vi "Can_Add.vi"(8 "error in (no error)":errorcluster, 11 "IB_Tree_Item_Proj_Folder in":refnum<class "IB_Tree_Item_Proj_Folder.lvclass">) -> (0 "error out":errorcluster, 2 "can add?":bool, 3 "IB_Tree_Item_Proj_Folder out":refnum<class "IB_Tree_Item_Proj_Folder.lvclass">)   [LabVIEW 2020, in "IB_Tree_Item_Proj_Folder.lvclass"]
uses:
  <vilib>/AppBuilder/IB_Classes/Tree_Item_Proj_Folder/IB_Tree_Item_Proj_Folder.lvclass
  <vilib>/AppBuilder/IB_Classes/Tree_Item_Proj_Folder/IB_Tree_Item_Proj_Folder.lvclass/IB_Tree_Item_Proj_Folder.ctl
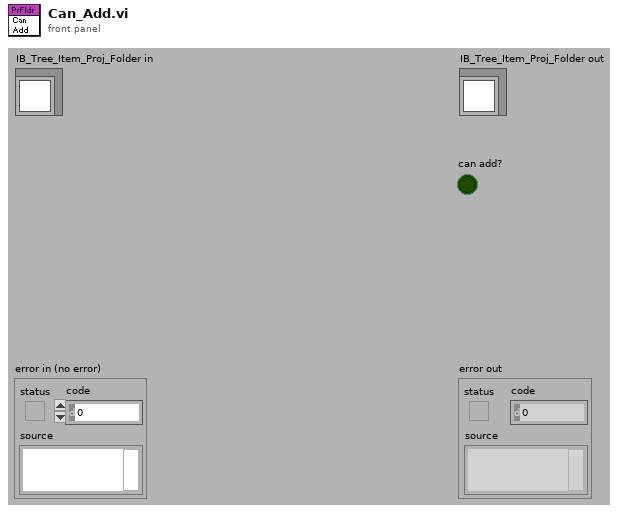
[diagram p1: front panel]
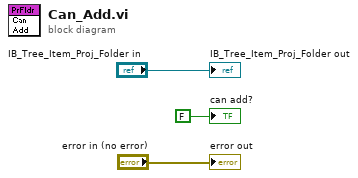
[diagram p0: block diagram]
diagram:
  "error out" <- "error in (no error)"
  "IB_Tree_Item_Proj_Folder out" <- "IB_Tree_Item_Proj_Folder in"
  "can add?" <- FALSE ("can add?")
